vi "DP-Construct DP vs Freq.vi"(0 "Data matrix":dbl[][](array[numeric]), 1 "Which DP":enum16{"2f1-f2", "f2-f1"}(ring), 11 "error in":errorcluster, 12 "L2 array":dbl[](array[numeric])) -> (13 "noise floor":T1(array[cluster]), 14 "IO Functions":T1(array[cluster]), 15 "error out":errorcluster)   [LabVIEW 2020]
panel:
  out "Numeric":i32
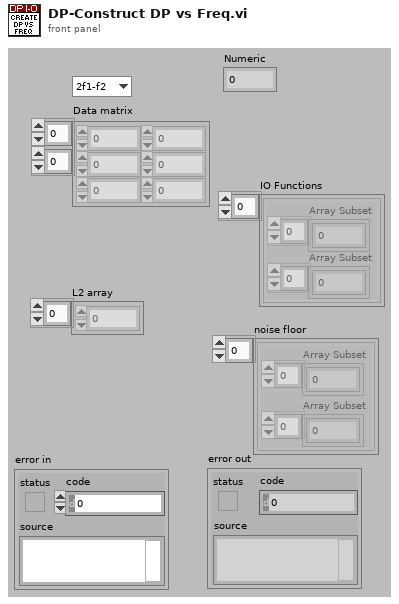
[diagram p1: front panel]
types:
  T1 = cluster{"Array Subset":dbl[], "Array Subset":dbl[]}[]
  T2 = cluster{"Array Subset":dbl[], "Array Subset":dbl[]}
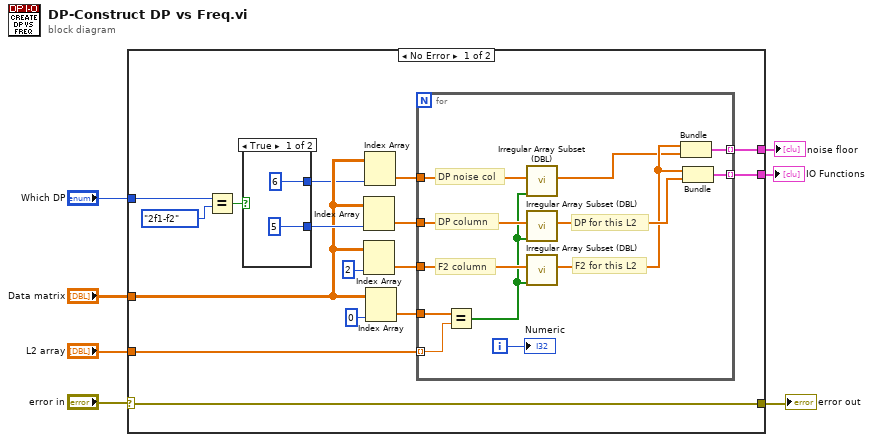
[diagram p0: block diagram]
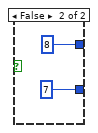
[diagram p2: hidden frame]
diagram:
  n1 = case shown="No Error" "error in" {
    selector: "error in" -> [w15 w40]
    tunnel: "Data matrix" -> [w11 _]
    tunnel: "L2 array" -> [w18 _]
    tunnel: "Which DP" -> [w17 _]
    tunnel: [w15 w40] -> w3
    tunnel: [w14 _] -> w2
    tunnel: [w8 _] -> w1
    frame No Error {
      n2 = Equal?(x=w17, y=enum16{"2f1-f2", "f2-f1"}."2f1-f2") -> (x = y?=w13:bool)
      n3 = case shown="True" w13 {
        tunnel: [5 ("disabled index (col)") 7 ("disabled index (col)")] -> w12
        tunnel: [6 ("disabled index (col)") 8 ("disabled index (col)")] -> w10
        frame True {
        }
        frame False {
        }
      }
      n4 = Index Array(array=w11, index (col)=w12) -> (element=w19:dbl[])  [unwired: 1 in]
      n5 = Index Array(array=w11, index (col)=2 ("index (row)")) -> (element=w21:dbl[])  [unwired: 1 in]
      n6 = Index Array(array=w11, index (col)=w10) -> (element=w9:dbl[])  [unwired: 1 in]
      n7 = Index Array(array=w11, index (col)=0 ("disabled index (col)")) -> (element=w22:dbl[])  [unwired: 1 in]
      n8 = for {
        tunnel: w22 -> [w39]
        tunnel: w21 -> [w38]
        tunnel: w19 -> [w37]
        tunnel: w18 -> [w32] mode=indexing
        tunnel: [w36] -> w14 mode=indexing
        tunnel: w9 -> [w35]
        tunnel: [w30] -> w8 mode=indexing
        i -> [w31]
        # "DP noise col"
        # "DP for this L2"
        # "F2 for this L2"
        # "DP column"
        # "F2 column"
        n9 = Equal?(x=w39, y=w32) -> (x = y?=w34:bool[])
        n10 = call "Irregular Array Subset (DBL).vi"("Mask"=w34, "Array"=w35) -> ("Array Subset"=w28:dbl[])  [unwired: 8 in, 1 out]
        n11 = call "Irregular Array Subset (DBL).vi"("Mask"=w34, "Array"=w37) -> ("Array Subset"=w33:dbl[])  [unwired: 8 in, 1 out]
        n12 = call "Irregular Array Subset (DBL).vi"("Mask"=w34, "Array"=w38) -> ("Array Subset"=w29:dbl[])  [unwired: 8 in, 1 out]
        n13 = Bundle("Array Subset"=w29, "Array Subset"=w28) -> (w30:T2)  [unwired: 1 in]
        n14 = Bundle("Array Subset"=w29, "Array Subset"=w33) -> (w36:T2)  [unwired: 1 in]
        "Numeric" <- w31
      }
    }
    frame Error {
    }
  }
  "error out" <- w3
  "IO Functions" <- w2
  "noise floor" <- w1
